vi "Main.vi"() -> ()   [LabVIEW 2016]
uses:
  EpubClass/EPUB.lvclass
  EpubClass/EPUB.lvclass/EPUB.ctl
panel:
  in  "线程":i32=4
  in  "输入类型":enum32{"IMG", "HTML", "MHT"}(radio)
  in  "大小过滤":i64=60000
  out "当前序号":i32
  out "EPUB数目":i32
  in  "工作临时目录":path=path "D:/Downloads"
  in  "Epub目录":path=path "D:/Downloads"
  out "水平刻度条":u32(slide) caption="创建EPUB..." scale=0.0..1.0
  out "inputPath":path caption="所选路径"
  in  "打开":bool
  in  "退出":bool
  in  "转换":bool
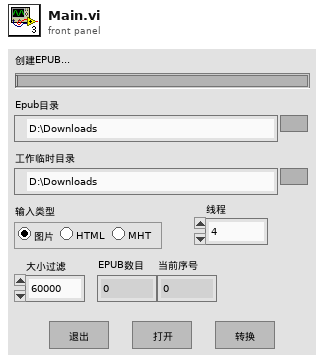
[diagram p1: front panel]
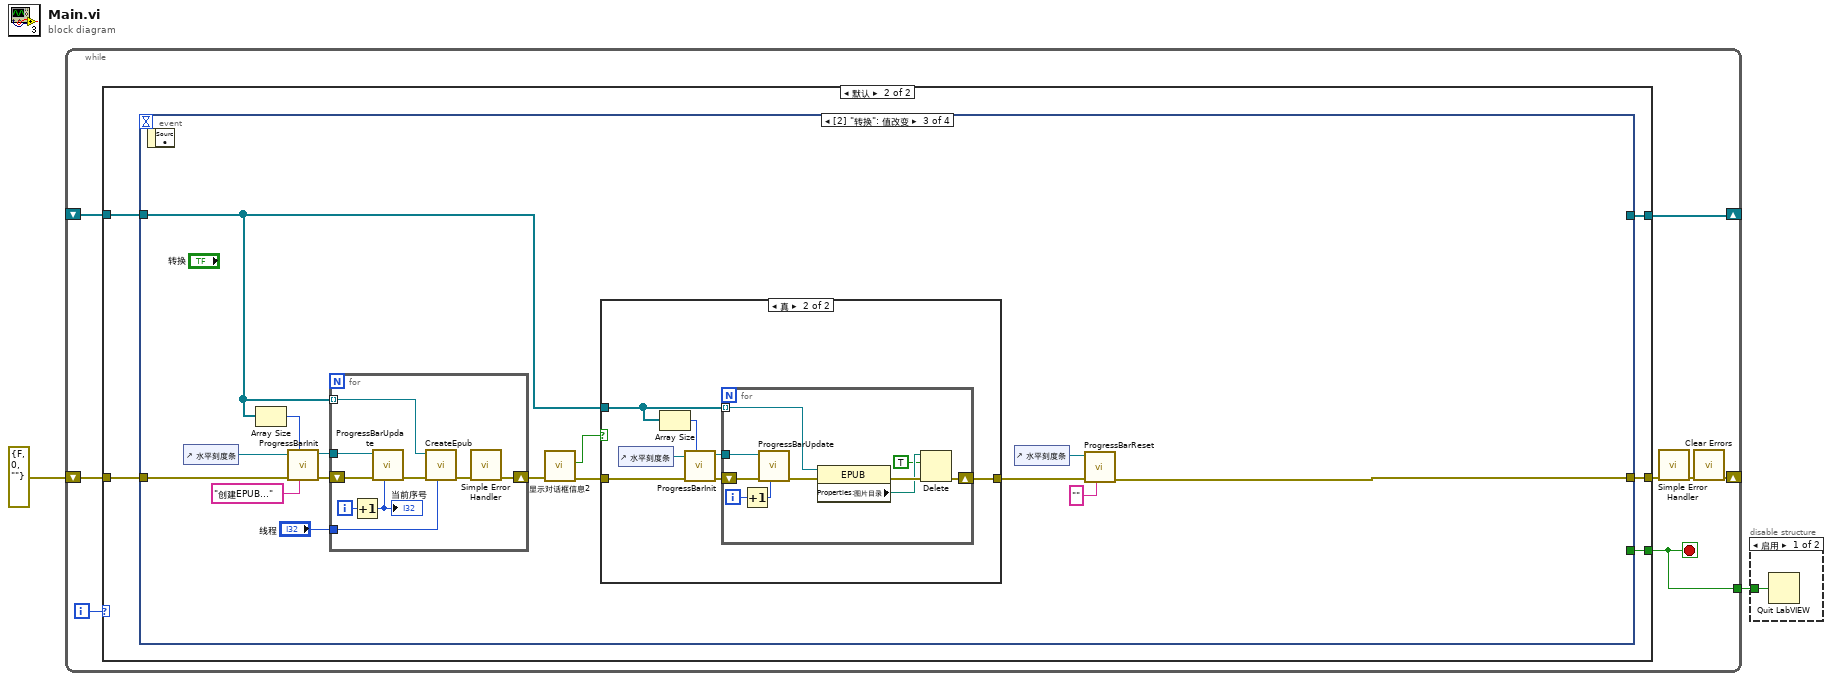
[diagram p0: block diagram]
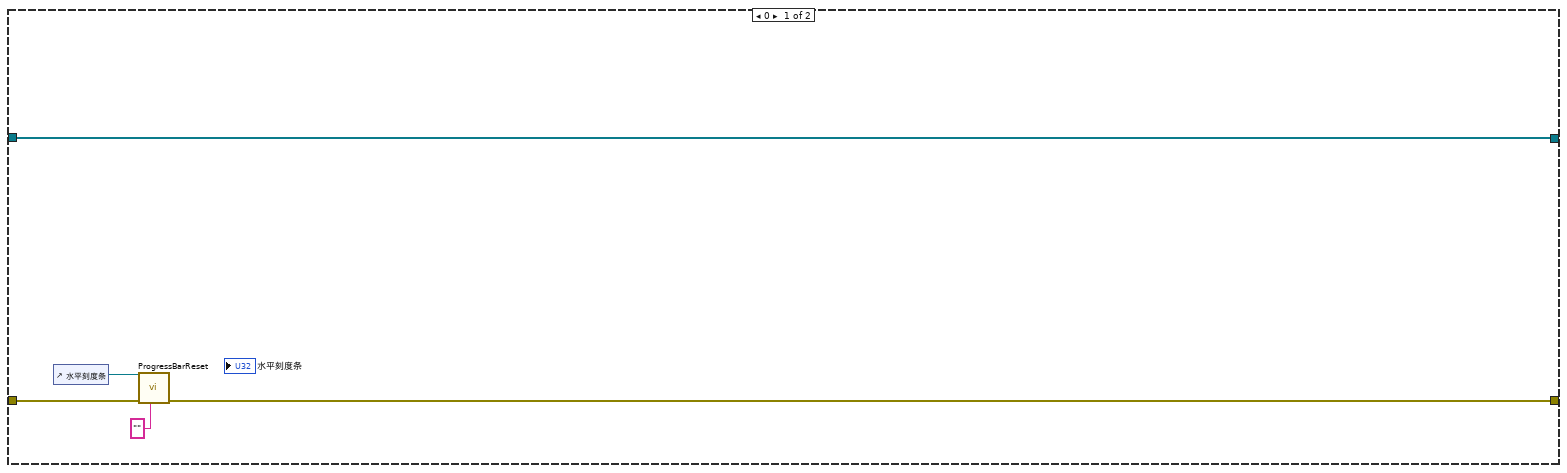
[diagram p3: hidden frame]
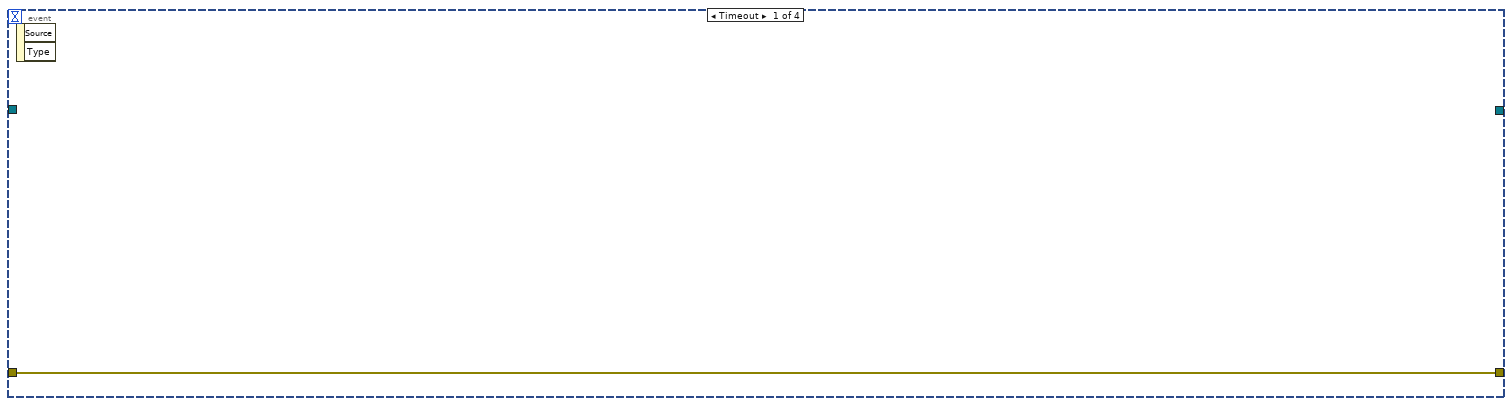
[diagram p4: hidden frame]
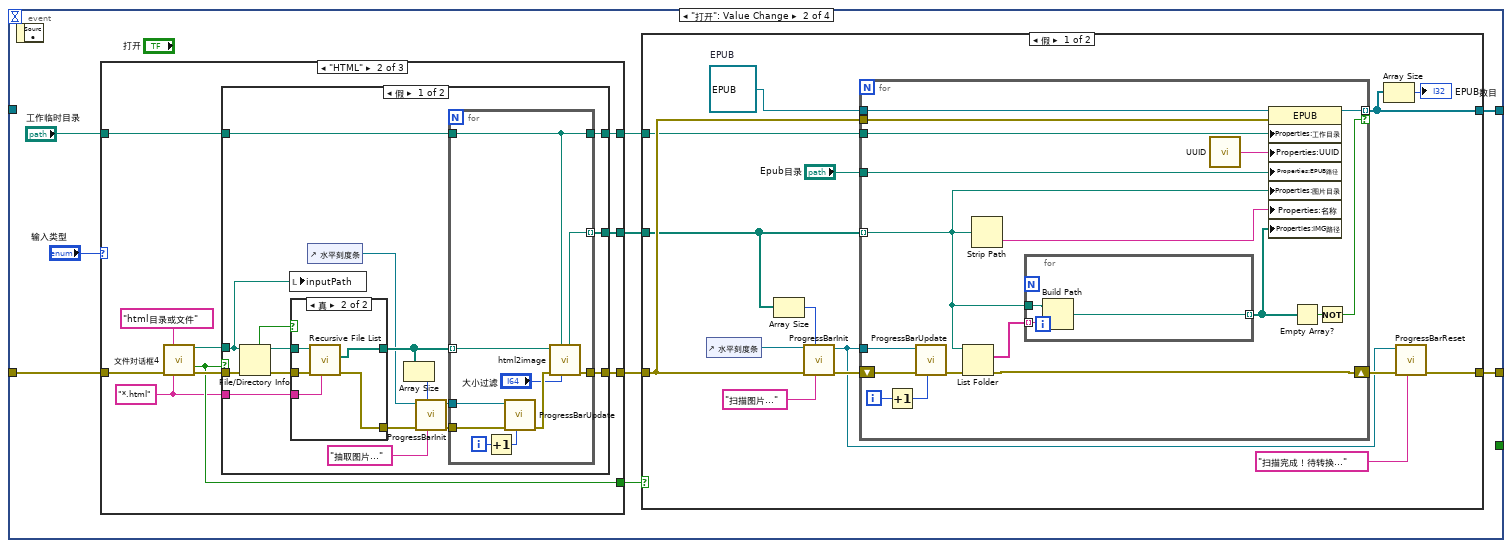
[diagram p5: hidden frame]
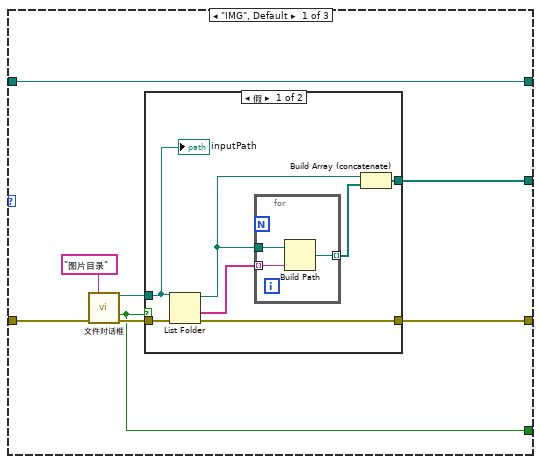
[diagram p6: hidden frame]
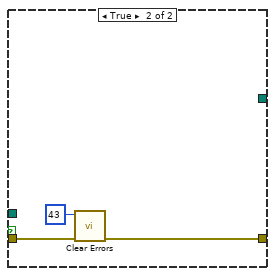
[diagram p7: hidden frame]
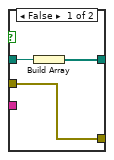
[diagram p8: hidden frame]
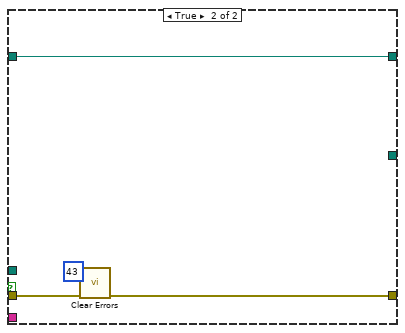
[diagram p9: hidden frame]
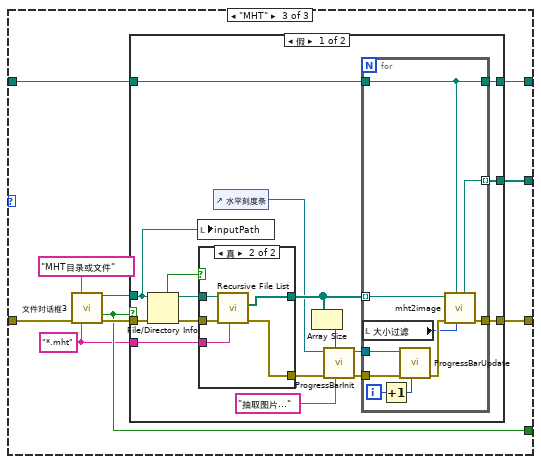
[diagram p10: hidden frame]
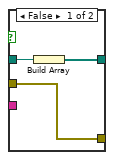
[diagram p11: hidden frame]
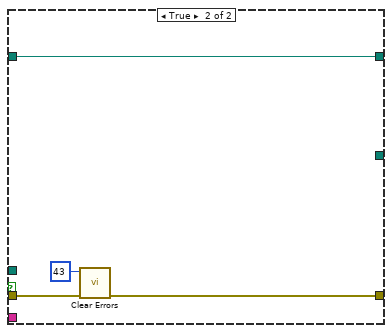
[diagram p12: hidden frame]
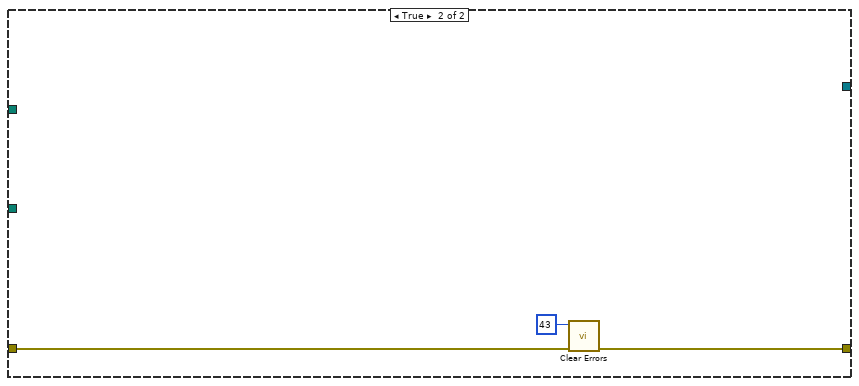
[diagram p13: hidden frame]
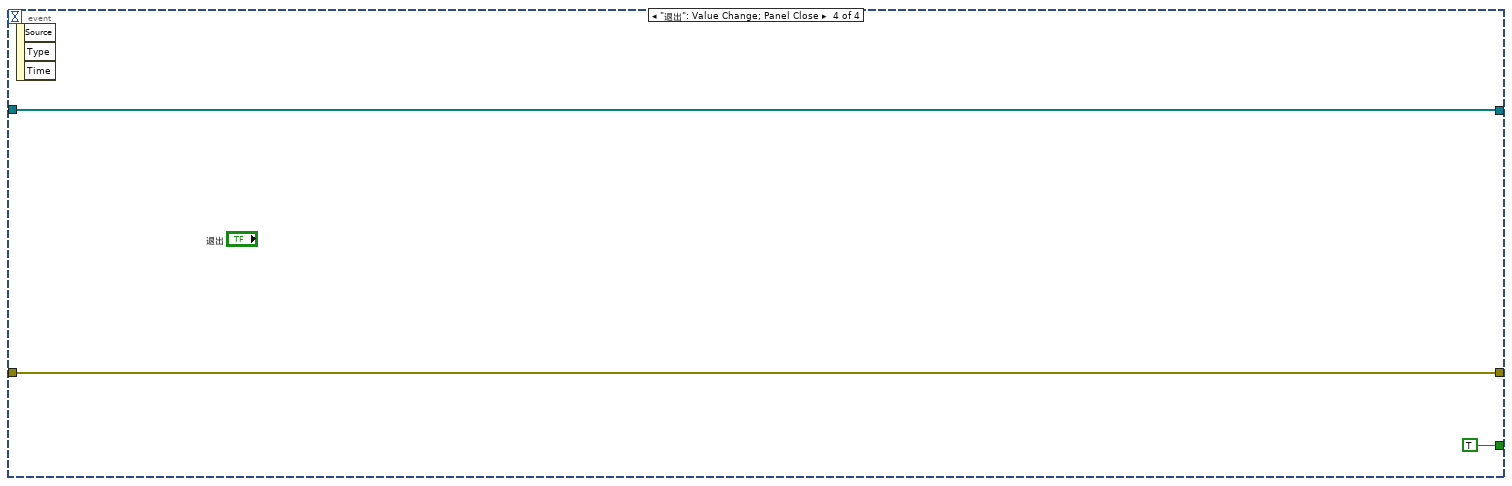
[diagram p15: hidden frame]
diagram:
  n1 = while {
    shift-right: [w3] -> _
    shift-left: errorcluster {"status"=FALSE, "code"=0, "source"=""} ("错误常量") -> [w9]
    shift-right: [w6] -> _
    shift-left: _ -> [w5]
    tunnel: [w4] -> w1
    i -> [w10]
    stop <- w4 stop-if-true
    n2 = case shown="默认" w10 {
      tunnel: w9 -> [w15 w20]
      tunnel: [w14 w19] -> w8
      tunnel: [_ w18] -> w4
      tunnel: [w11 w17] -> w6
      tunnel: w5 -> [w11 w16]
      frame 0 {
        # "初始化"
        n3 = control-ref of="水平刻度条"() -> (w13:refnum<vi>)
        n4 = call <vilib>:"ProgressBarReset.vi"("Title"="", "Error in"=w15, "ProgressBar"=w13) -> ("Error out"=w14:errorcluster)  [unwired: 7 in, 1 out]
      }
      frame Default {
        n5 = event shown="[2] \"转换\": 值改变" {
          selector: _ -> [_ _ _ _]
          dyn-events: _ -> [_ _ _ _]
          timeout: _ -> [_ _ _ _]
          tunnel: w20 -> [w21 w30 w203 w232]
          tunnel: [w21 w28 w195 w232] -> w19
          tunnel: [_ _ _ TRUE] -> w18
          tunnel: [_ w26 _ w231] -> w17
          tunnel: w16 -> [_ _ w191 w231]
          event Timeout {
            n6 = event-data() -> ()  [unwired: 1 in, 2 out]
          }
          event "打开": Value Change {
            n7 = event-data() -> ()  [unwired: 1 in, 1 out]
            n8 = case shown="\"HTML\"" "输入类型" {
              tunnel: w30 -> [w38 w61 w110]
              tunnel: [w35 w60 w109] -> w29
              tunnel: [w32 w54 w103] -> w27
              tunnel: [w33 w59 w108] -> w25
              tunnel: [w31 w58 w107] -> w23
              tunnel: "工作临时目录" -> [w31 w57 w106]
              frame "IMG", Default {
                n9 = call "文件对话框"("prompt"="图片目录", "error in"=w38) -> ("selected path"=w36:path, "cancelled"=w32:bool, "error out"=w34:errorcluster)  [unwired: 10 in, 1 out]
                n10 = case shown="假" w32 {
                  tunnel: w36 -> [w42 _]
                  tunnel: [w41 w50] -> w35
                  tunnel: w34 -> [w40 w51]
                  tunnel: [w39 _] -> w33
                  frame False {
                    n11 = List Folder(path=w42, error in=w40) -> (path out=w43:path, folder names=w45:string[], error out=w41:errorcluster)  [unwired: 2 in, 1 out]
                    n12 = for {
                      tunnel: w45 -> [w48] mode=indexing
                      tunnel: w43 -> [w47]
                      tunnel: [w46] -> w44 mode=indexing
                      n13 = Build Path(base path=w47, name or relative path=w48) -> (appended path=w46:path)
                    }
                    n14 = Build Array (concatenate)(w43, w44) -> (w39:path[])
                    "inputPath" <- w42
                  }
                  frame True {
                    n15 = call <vilib>:"Clear Errors.vi"("error in (no error)"=w51, "specific error code to clear (0: all)"=43) -> ("error out"=w50:errorcluster)  [unwired: 4 in, 1 out]
                  }
                }
              }
              frame "HTML" {
                w52 = "*.html" ("pattern (all files)")
                n16 = call "文件对话框4"("prompt"="html目录或文件", "error in"=w61, "pattern (all files)"=w52) -> ("selected path"=w53:path, "cancelled"=w54:bool, "error out"=w56:errorcluster)  [unwired: 9 in, 1 out]
                n17 = case shown="假" w54 {
                  tunnel: [w78 w99] -> w60
                  tunnel: [w77 _] -> w59
                  tunnel: [w76 w97] -> w58
                  tunnel: w57 -> [w75 w97]
                  tunnel: w56 -> [w74 w100]
                  tunnel: w53 -> [w69 _]
                  tunnel: w52 -> [w68 _]
                  frame False {
                    n18 = File/Directory Info(path=w69, error in=w74) -> (path out=w71:path, directory=w70:bool, error out=w72:errorcluster)  [unwired: 4 out]
                    n19 = local write "inputPath"(w69) -> ()
                    n20 = case shown="真" w70 {
                      tunnel: [w81 w86] -> w73
                      tunnel: w72 -> [w81 w85]
                      tunnel: w71 -> [w80 w84]
                      tunnel: [w79 w83] -> w65
                      tunnel: w68 -> [_ w82]
                      frame False {
                        n21 = Build Array(w80) -> (w79:path[])
                      }
                      frame True {
                        n22 = call <vilib>:"Recursive File List.vi"("pattern"=w82, "error in (no error)"=w85, "Folder Path"=w84) -> ("error out"=w86:errorcluster, "All Files in Dir"=w83:path[])  [unwired: 4 in, 3 out]
                      }
                    }
                    n23 = control-ref of="水平刻度条"() -> (w62:refnum<vi>)
                    n24 = Array Size(array=w65) -> (size(s)=w66:i32)
                    n25 = call <vilib>:"ProgressBarInit.vi"("Title"="抽取图片...", "Maximum"=w66, "Error in"=w73, "ProgressBar"=w62) -> ("Error out"=w67:errorcluster, "ProgressBarO"=w64:refnum<vi>)  [unwired: 6 in]
                    n26 = for {
                      tunnel: [w94] -> w77 mode=indexing
                      tunnel: [w93] -> w76
                      tunnel: w75 -> [w93]
                      tunnel: w67 -> [w96]
                      tunnel: [w95] -> w78
                      tunnel: w65 -> [w92] mode=indexing
                      tunnel: w64 -> [w90]
                      i -> [w89]
                      n27 = Increment(x=w89) -> (x+1=w88:i32)
                      n28 = call <vilib>:"ProgressBarUpdate.vi"("Value"=w88, "Error in"=w96, "ProgressBar"=w90) -> ("Error out"=w91:errorcluster)  [unwired: 7 in, 1 out]
                      n29 = call "html2image.vi"("size"="大小过滤", "IMGPath"=w93, "Error in"=w91, "html"=w92) -> ("Error out"=w95:errorcluster, "ImagePath"=w94:path)  [unwired: 5 in, 1 out]
                    }
                  }
                  frame True {
                    n30 = call <vilib>:"Clear Errors.vi"("error in (no error)"=w100, "specific error code to clear (0: all)"=43) -> ("error out"=w99:errorcluster)  [unwired: 4 in, 1 out]
                  }
                }
              }
              frame "MHT" {
                w101 = "*.mht" ("pattern (all files)")
                n31 = call "文件对话框3"("prompt"="MHT目录或文件", "error in"=w110, "pattern (all files)"=w101) -> ("selected path"=w102:path, "cancelled"=w103:bool, "error out"=w105:errorcluster)  [unwired: 9 in, 1 out]
                n32 = case shown="假" w103 {
                  tunnel: [w127 w148] -> w109
                  tunnel: [w126 _] -> w108
                  tunnel: [w125 w146] -> w107
                  tunnel: w106 -> [w124 w146]
                  tunnel: w105 -> [w123 w149]
                  tunnel: w102 -> [w118 _]
                  tunnel: w101 -> [w117 _]
                  frame False {
                    n33 = File/Directory Info(path=w118, error in=w123) -> (path out=w120:path, directory=w119:bool, error out=w121:errorcluster)  [unwired: 4 out]
                    n34 = local write "inputPath"(w118) -> ()
                    n35 = case shown="真" w119 {
                      tunnel: [w130 w135] -> w122
                      tunnel: w121 -> [w130 w134]
                      tunnel: w120 -> [w129 w133]
                      tunnel: [w128 w132] -> w114
                      tunnel: w117 -> [_ w131]
                      frame False {
                        n36 = Build Array(w129) -> (w128:path[])
                      }
                      frame True {
                        n37 = call <vilib>:"Recursive File List.vi"("pattern"=w131, "error in (no error)"=w134, "Folder Path"=w133) -> ("error out"=w135:errorcluster, "All Files in Dir"=w132:path[])  [unwired: 4 in, 3 out]
                      }
                    }
                    n38 = control-ref of="水平刻度条"() -> (w111:refnum<vi>)
                    n39 = Array Size(array=w114) -> (size(s)=w115:i32)
                    n40 = call <vilib>:"ProgressBarInit.vi"("Title"="抽取图片...", "Maximum"=w115, "Error in"=w122, "ProgressBar"=w111) -> ("Error out"=w116:errorcluster, "ProgressBarO"=w113:refnum<vi>)  [unwired: 6 in]
                    n41 = for {
                      tunnel: [w143] -> w126 mode=indexing
                      tunnel: [w142] -> w125
                      tunnel: w124 -> [w142]
                      tunnel: w116 -> [w145]
                      tunnel: [w144] -> w127
                      tunnel: w114 -> [w141] mode=indexing
                      tunnel: w113 -> [w139]
                      i -> [w138]
                      n42 = local read "大小过滤"() -> (w136:i64)
                      n43 = Increment(x=w138) -> (x+1=w137:i32)
                      n44 = call <vilib>:"ProgressBarUpdate.vi"("Value"=w137, "Error in"=w145, "ProgressBar"=w139) -> ("Error out"=w140:errorcluster)  [unwired: 7 in, 1 out]
                      n45 = call "mht2image.vi"("size"=w136, "IMGPath"=w142, "Error in"=w140, "mht"=w141) -> ("Error out"=w144:errorcluster, "ImagePath"=w143:path)  [unwired: 5 in, 1 out]
                    }
                  }
                  frame True {
                    n46 = call <vilib>:"Clear Errors.vi"("error in (no error)"=w149, "specific error code to clear (0: all)"=43) -> ("error out"=w148:errorcluster)  [unwired: 4 in, 1 out]
                  }
                }
              }
            }
            n47 = case shown="假" w27 {
              tunnel: w29 -> [w156 w188]
              tunnel: [w154 w187] -> w28
              tunnel: [w157 _] -> w26
              tunnel: w25 -> [w155 _]
              tunnel: w23 -> [w150 _]
              frame False {
                w151 = refnum<class "EPUB.lvclass"> refnum  # EPUB
                n48 = control-ref of="水平刻度条"() -> (w159:refnum<vi>)
                n49 = Array Size(array=w155) -> (size(s)=w162:i32)
                n50 = call <vilib>:"ProgressBarInit.vi"("Title"="扫描图片...", "Maximum"=w162, "Error in"=w156, "ProgressBar"=w159) -> ("Error out"=w161:errorcluster, "ProgressBarO"=w153:refnum<vi>)  [unwired: 6 in]
                n51 = for {
                  shift-right: [w165] -> w164
                  shift-left: w161 -> [w182]
                  tunnel: w151 -> [w181]
                  tunnel: w156 -> [w172]
                  tunnel: [w175] -> w157 mode=indexing if=w173
                  tunnel: "Epub目录" -> [w171]
                  tunnel: w153 -> [w179]
                  tunnel: w155 -> [w167] mode=indexing
                  tunnel: w150 -> [w169]
                  i -> [w178]
                  n52 = Increment(x=w178) -> (x+1=w177:i32)
                  n53 = call <vilib>:"ProgressBarUpdate.vi"("Value"=w177, "Error in"=w182, "ProgressBar"=w179) -> ("Error out"=w180:errorcluster)  [unwired: 7 in, 1 out]
                  n54 = List Folder(path=w167, error in=w180) -> (filenames=w176:string[], error out=w165:errorcluster)  [unwired: 2 in, 2 out]
                  n55 = Strip Path(path=w167) -> (name=w168:string)  [unwired: 1 out]
                  n56 = for {
                    tunnel: w167 -> [w185]
                    tunnel: w176 -> [w184] mode=indexing
                    tunnel: [w183] -> w166 mode=indexing
                    n57 = Build Path(base path=w185, name or relative path=w184) -> (appended path=w183:path)
                  }
                  n58 = call "UUID.vi"() -> ("UUID"=w170:string)  [unwired: 1 in]
                  n59 = property class="EPUB"(reference=w181, error in=w172, "Properties:工作目录"=w169, "Properties:UUID"=w170, "Properties:EPUB路径"=w171, "Properties:图片目录"=w167, "Properties:名称"=w168, "Properties:IMG路径"=w166) -> (reference out=w175:refnum<class "EPUB.lvclass">)  [unwired: 1 out]
                  n60 = Empty Array?(array=w166) -> (empty?=w174:bool)
                  n61 = Not(x=w174) -> (.not. x?=w173:bool)
                }
                n62 = Array Size(array=w157) -> (size(s)=→"EPUB数目":i32)
                n63 = call <vilib>:"ProgressBarReset.vi"("Title"="扫描完成！待转换...", "Error in"=w164, "ProgressBar"=w153) -> ("Error out"=w154:errorcluster)  [unwired: 7 in, 1 out]
              }
              frame True {
                n64 = call <vilib>:"Clear Errors.vi"("error in (no error)"=w188, "specific error code to clear (0: all)"=43) -> ("error out"=w187:errorcluster)  [unwired: 4 in, 1 out]
              }
            }
          }
          event "转换": Value Change {
            n65 = event-data() -> ()  [unwired: 1 in, 1 out]
            n66 = control-ref of="水平刻度条"() -> (w200:refnum<vi>)
            n67 = Array Size(array=w191) -> (size(s)=w196:i32)
            n68 = call <vilib>:"ProgressBarInit.vi"("Title"="创建EPUB...", "Maximum"=w196, "Error in"=w203, "ProgressBar"=w200) -> ("Error out"=w202:errorcluster, "ProgressBarO"=w199:refnum<vi>)  [unwired: 6 in]
            n69 = for {
              shift-right: [w224] -> w198
              shift-left: w202 -> [w230]
              tunnel: w199 -> [w228]
              tunnel: w191 -> [w225] mode=indexing
              tunnel: "线程" -> [w222]
              i -> [w227]
              n70 = Increment(x=w227) -> (x+1=w226:i32)
              "当前序号" <- w226
              n71 = call <vilib>:"ProgressBarUpdate.vi"("Value"=w226, "Error in"=w230, "ProgressBar"=w228) -> ("Error out"=w229:errorcluster)  [unwired: 7 in, 1 out]
              n72 = call "CreateEpub.vi"("线程"=w222, "error in (no error)"=w229, "EPUB 输入"=w225) -> ("error out"=w223:errorcluster)  [unwired: 7 in, 1 out]
              n73 = call <vilib>:"Simple Error Handler.vi"("error in (no error)"=w223) -> ("error out"=w224:errorcluster)  [unwired: 4 in, 4 out]
            }
            n74 = call "显示对话框信息2"("error in (no error)"=w198) -> ("error out"=w192:errorcluster, "确定"=w190:bool)  [unwired: 9 in]
            n75 = case shown="真" w190 {
              tunnel: [w204 w210] -> w197
              tunnel: w192 -> [w204 w211]
              tunnel: w191 -> [_ w206]
              frame False {
              }
              frame True {
                n76 = control-ref of="水平刻度条"() -> (w205:refnum<vi>)
                n77 = Array Size(array=w206) -> (size(s)=w207:i32)
                n78 = call <vilib>:"ProgressBarInit.vi"("Maximum"=w207, "Error in"=w211, "ProgressBar"=w205) -> ("Error out"=w209:errorcluster, "ProgressBarO"=w208:refnum<vi>)  [unwired: 7 in]
                n79 = for {
                  shift-right: [w221] -> w210
                  shift-left: w209 -> [w220]
                  tunnel: w206 -> [w218] mode=indexing
                  tunnel: w208 -> [w214]
                  i -> [w213]
                  n80 = Increment(x=w213) -> (x+1=w212:i32)
                  n81 = call <vilib>:"ProgressBarUpdate.vi"("Value"=w212, "Error in"=w220, "ProgressBar"=w214) -> ("Error out"=w215:errorcluster)  [unwired: 7 in, 1 out]
                  n82 = property class="EPUB"(reference=w218, error in=w215) -> (error out=w219:errorcluster, "Properties:图片目录"=w217:path)  [unwired: 1 out]
                  n83 = Delete(path (use dialog)=w217, entire hierarchy (F)=TRUE ("整个层次结构(F)"), error in=w219) -> (error out=w221:errorcluster)  [unwired: 2 in, 2 out]
                }
              }
            }
            n84 = control-ref of="水平刻度条"() -> (w194:refnum<vi>)
            n85 = call <vilib>:"ProgressBarReset.vi"("Title"="", "Error in"=w197, "ProgressBar"=w194) -> ("Error out"=w195:errorcluster)  [unwired: 7 in, 1 out]
          }
          event "退出": Value Change; Panel Close {
            n86 = event-data() -> ()  [unwired: 1 in, 3 out]
          }
        }
      }
    }
    n87 = call <vilib>:"Simple Error Handler.vi"("error in (no error)"=w8) -> ("error out"=w7:errorcluster)  [unwired: 4 in, 4 out]
    n88 = call <vilib>:"Clear Errors.vi"("error in (no error)"=w7) -> ("error out"=w3:errorcluster)  [unwired: 5 in, 1 out]
  }
  n89 = disable-structure shown="启用" {
    disable-tunnel: w1 -> [w234 _]
    frame Enabled {
      n90 = Quit LabVIEW(quit? (T)=w234) -> ()
    }
    frame Disabled {
    }
  }
